vi "Instrument.Lockin.GetPublicEvents.vi"(8 "error in (no error)":errorcluster, 11 "Instrument.Lockin in":refnum<class "Instrument.Lockin.lvclass">) -> (0 "error out":errorcluster, 3 "Instrument.Lockin out":refnum<class "Instrument.Lockin.lvclass">)   [LabVIEW 2019, in "Instrument.Lockin.lvclass"]
uses:
  Instrument.Lockin.lvclass
  Typedefs/PublicEvents--Instrument.Lockin.getAO.ctl
  Typedefs/PublicEvents--Cluster.ctl
panel:
  out "Lockin.Public Events":T1
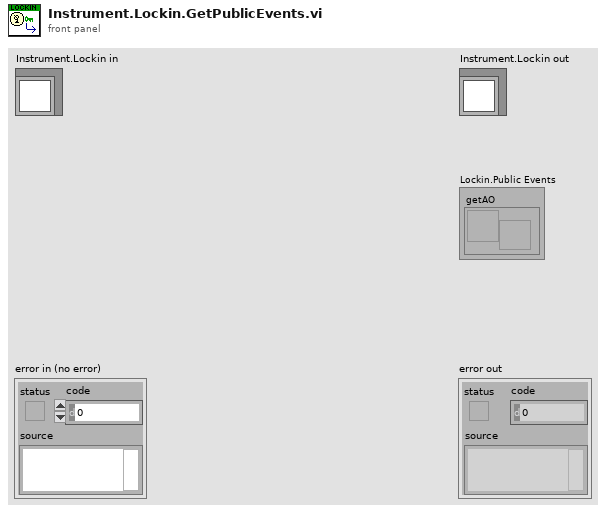
[diagram p1: front panel]
types:
  T1 = typedef "Instrument.Lockin.lvclass/PublicEvents--Cluster.ctl" = cluster{"getAO":refnum<user-event>}
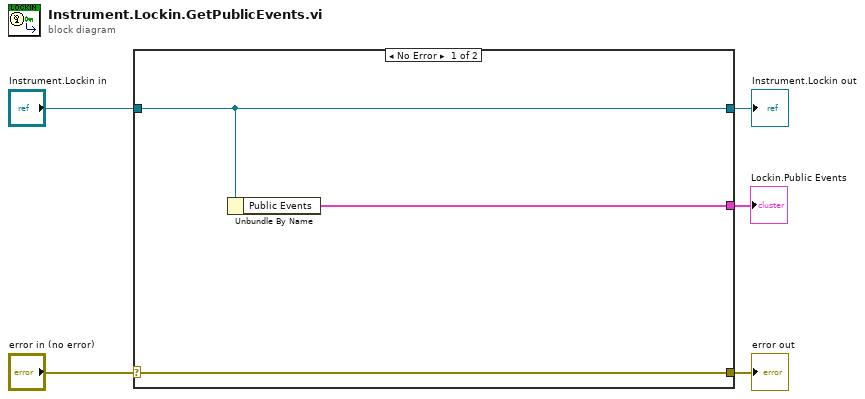
[diagram p0: block diagram]
diagram:
  n1 = case shown="No Error" "error in (no error)" {
    selector: "error in (no error)" -> [w8 w10]
    tunnel: [w8 w10] -> w4
    tunnel: [w7 w9] -> w2
    tunnel: "Instrument.Lockin in" -> [w7 w9]
    tunnel: [w6 _] -> w1
    frame No Error {
      n2 = Unbundle By Name(w7) -> ("Public Events"=w6:T1)
    }
    frame Error {
    }
  }
  "error out" <- w4
  "Instrument.Lockin out" <- w2
  "Lockin.Public Events" <- w1
